vi "QSM - Add State(s) to Front.vi"(6 "QSM":T1={"Invalid Option"=enum."Ignore", "QSM"=refnum}, 7 "Act? (T)":bool=TRUE, 8 "error in (no error)":errorcluster, 11 "State(s)":string) -> (0 "error out":errorcluster)   [LabVIEW 2014]
doc: "This VI Add States to the Front of the Queue\n\nDataEtc Copyright (c) 2013"
uses:
  TypeDef/QSM - STYP.ctl
  TypeDef/Invalid Option - STYP.ctl
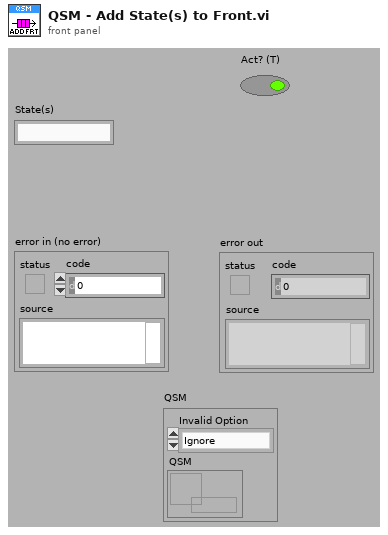
[diagram p1: front panel]
types:
  T1 = typedef "QSM - STYP.ctl" = cluster{"Invalid Option":T2, "QSM":refnum<queue>}
  T2 = typedef "Invalid Option - STYP.ctl" = enum16{"Dialog", "Error", "Ignore"}
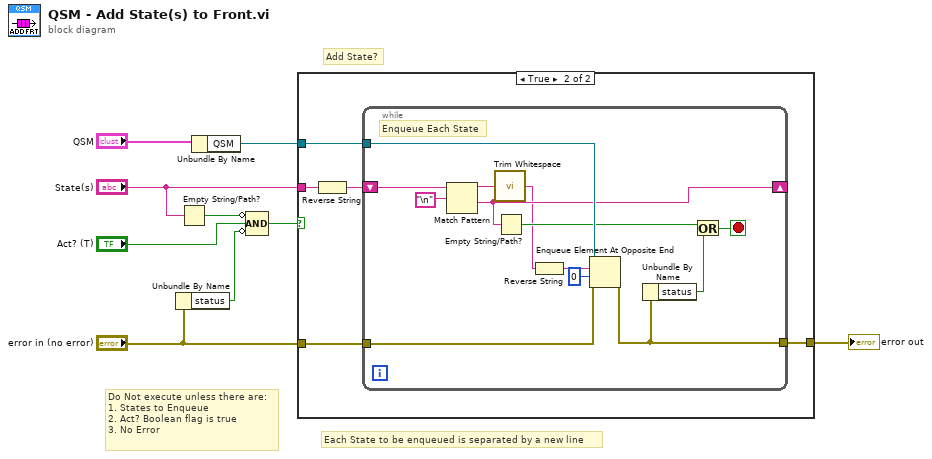
[diagram p0: block diagram]
diagram:
  # "Do Not execute unless there are:\n1. States to Enqueue\n2. Act? Boolean flag is true\n3. No Error"
  # "Each State to be enqueued is separated by a new line"
  # "Add State?"
  n1 = Unbundle By Name("error in (no error)") -> ("status"=w6:bool)
  n2 = Empty String/Path?(string/path="State(s)") -> (empty?=w8:bool)
  n3 = Unbundle By Name("QSM") -> ("QSM"=w2:refnum<queue>)
  n4 = Compound Arithmetic op=AND(invert w8, "Act? (T)", invert w6) -> (w5:bool)
  n5 = case shown="True" w5 {
    tunnel: "error in (no error)" -> [w10 w15]
    tunnel: "State(s)" -> [_ w12]
    tunnel: w2 -> [_ w14]
    tunnel: [w10 w13] -> w1
    frame False {
    }
    frame True {
      n6 = Reverse String(1:w12) -> (0:w11:string)
      n7 = while {
        tunnel: w15 -> [w27]
        tunnel: w14 -> [w28]
        shift-right: [w22] -> _
        shift-left: w11 -> [w26]
        tunnel: [w21] -> w13
        stop <- w18 stop-if-true
        # "Enqueue Each State"
        n8 = Match Pattern(string=w26, regular expression="\n") -> (before substring=w24:string, after substring=w22:string)  [unwired: 3 out]
        n9 = call <vilib>:"Trim Whitespace.vi"("string"=w24) -> ("trimmed string"=w17:string)  [unwired: 1 in]
        n10 = Empty String/Path?(string/path=w22) -> (empty?=w20:bool)
        n11 = Reverse String(1:w17) -> (0:w16:string)
        n12 = Enqueue Element At Opposite End(queue=w28, element=w16, timeout in ms (-1)=0, error in (no error)=w27) -> (error out=w21:errorcluster)  [unwired: 2 out]
        n13 = Unbundle By Name(w21) -> ("status"=w19:bool)
        n14 = Or(x=w20, y=w19) -> (x .or. y?=w18:bool)
      }
    }
  }
  "error out" <- w1
